vi "save_time_average.vi"(7 "stimulation type enum":T1, 8 "error in (no error)":errorcluster, 9 "base name":string, 10 "folder path":path, 11 "DataCollectionMG091001IntrinsicImaging in":refnum<class "DataCollectionMG091001IntrinsicImaging.lvclass">) -> (0 "error out":errorcluster, 3 "DataCollectionMG091001IntrinsicImaging out":refnum<class "DataCollectionMG091001IntrinsicImaging.lvclass">)   [LabVIEW 2010, in "DataCollectionMG091001IntrinsicImaging.lvclass"]
uses:
  DataCollectionMG091001IntrinsicImaging.lvclass
  sweep_part_enum.ctl
  common/classes/ImageCollection/ImageCollection/ImageCollection.lvclass
  DataCollectionMG091001IntrinsicImaging.lvclass/DataCollectionMG091001IntrinsicImaging.ctl
  common/classes/ImageCollection/ImageCollection/add_mode_enum.ctl
  common/classes/ErrorController/ErrorController/class_data.vi
  common/classes/ErrorController/ErrorController/ErrorController.lvclass
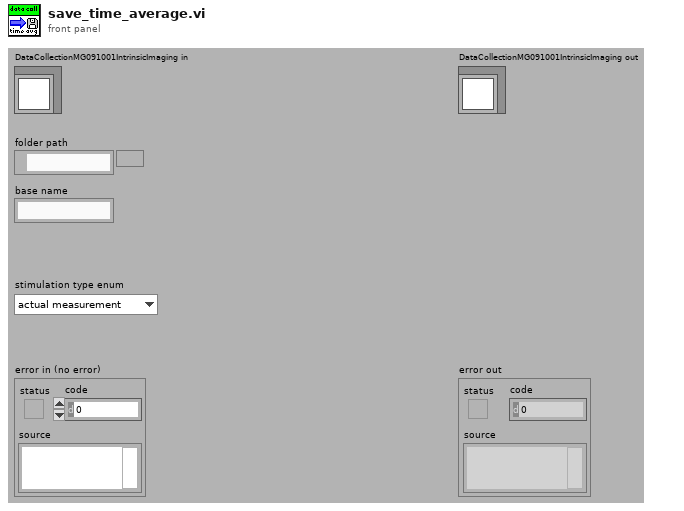
[diagram p1: front panel]
types:
  T1 = typedef "DataCollectionMG091001IntrinsicImaging.lvclass/sweep_part_enum.ctl" = enum16{"actual measurement", "control"}
  T2 = typedef "ImageCollection.lvclass/add_mode_enum.ctl" = enum16{"instance", "copy"}
  T3 = typedef "DataCollectionMG091001IntrinsicImaging.lvclass/individual_sweeps_saving_enum.ctl" = enum32{"autosave sweeps on the fly", "save individual sweeps", "don't save individual sweeps"}
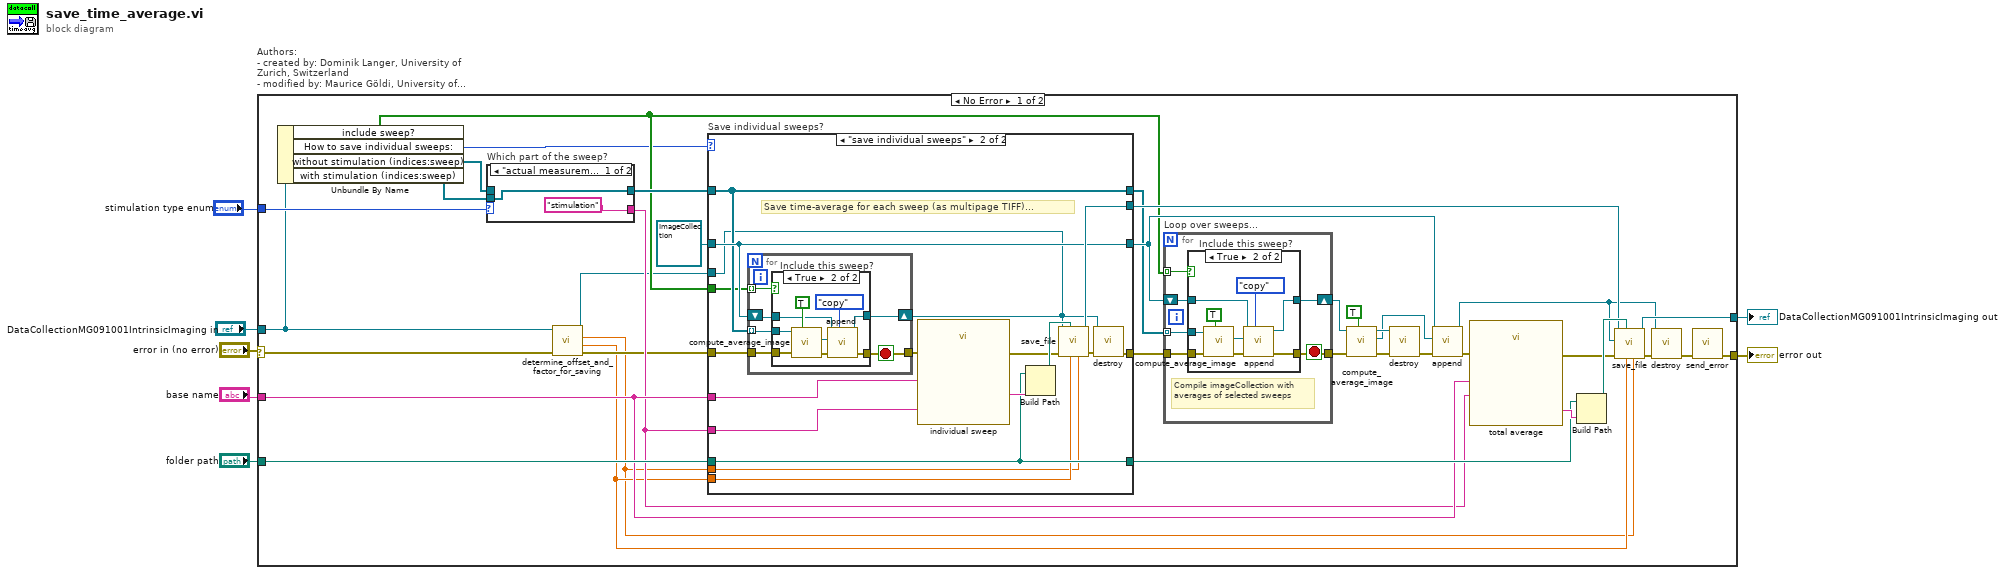
[diagram p0: block diagram]
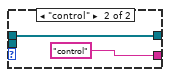
[diagram p2: hidden frame]
diagram:
  n1 = case "Authors: \n- created by: Dominik Langer, University of Zurich, Switzerland\n- modified by: Maurice Göldi, University of Zurich, Switzerland\n- modified by: Dominik Langer, University of Zurich, Switzerland" shown="No Error" "error in (no error)" {
    selector: "error in (no error)" -> [w15 w107]
    tunnel: [w16 w107] -> w6
    tunnel: [w44 w106] -> w4
    tunnel: "DataCollectionMG091001IntrinsicImaging in" -> [w13 w106]
    tunnel: "base name" -> [w26 _]
    tunnel: "folder path" -> [w43 _]
    tunnel: "stimulation type enum" -> [w22 _]
    frame No Error {
      n2 = Unbundle By Name(w13) -> ("include sweep?"=w19:bool[], "How to save individual sweeps:"=w18:T3, "without stimulation (indices:sweep)"=w23:refnum<class "ImageCollection.lvclass">[], "with stimulation (indices:sweep)"=w24:refnum<class "ImageCollection.lvclass">[])
      n3 = case "Which part of the sweep?" shown="\"actual measurement\", Default" w22 {
        tunnel: w23 -> [_ w48]
        tunnel: w24 -> [w46 _]
        tunnel: [w46 w48] -> w21
        tunnel: ["stimulation" "control"] -> w20
        frame "actual measurement", Default {
        }
        frame "control" {
        }
      }
      n4 = call-dynamic "determine_offset_and_factor_for_saving.vi"("error in (no error)"=w15, "DataCollectionMG091001IntrinsicImaging in"=w13) -> ("error out"=w14:errorcluster, "factor"=w9:dbl, "offset"=w8:dbl, "DataCollectionMG091001IntrinsicImaging out"=w12:refnum<class "DataCollectionMG091001IntrinsicImaging.lvclass">)  [unwired: 6 in]
      n5 = case "Save individual sweeps?" shown="\"save individual sweeps\"" w18 {
        tunnel: w14 -> [w70 w88]
        tunnel: w12 -> [w69 w75]
        tunnel: w21 -> [w66 w77]
        tunnel: [w69 w85] -> w29
        tunnel: w26 -> [_ w82]
        tunnel: w20 -> [_ w81]
        tunnel: w43 -> [w68 w79]
        tunnel: [w70 w80] -> w31
        tunnel: [w68 w79] -> w30
        tunnel: refnum<class "ImageCollection.lvclass"> refnum ("ImageCollection.lvclass") -> [w67 w78]
        tunnel: [w67 w78] -> w28
        tunnel: [w66 w77] -> w27
        tunnel: w19 -> [_ w76]
        tunnel: w9 -> [_ w72]
        tunnel: w8 -> [_ w71]
        frame Default {
        }
        frame "save individual sweeps" {
          # "Save time-average for each sweep (as multipage TIFF)..."
          n6 = for {
            tunnel: w77 -> [w94] mode=indexing
            shift-right: [w91] -> w73
            shift-left: w78 -> [w92]
            tunnel: w76 -> [w90] mode=indexing
            tunnel: w88 -> [w93]
            tunnel: [w89] -> w87
            stop <- w89 stop-if-true
            n7 = case "Include this sweep?" shown="True" w90 {
              tunnel: w94 -> [_ w105]
              tunnel: w93 -> [w96 w103]
              tunnel: w92 -> [w95 w101]
              tunnel: [w95 w99] -> w91
              tunnel: [w96 w97] -> w89
              frame False {
              }
              frame True {
                n8 = call-dynamic "compute_average_image.vi"("all?"=TRUE, "error in (no error)"=w103, "ImageCollection in"=w105) -> ("error out"=w102:errorcluster, "averaged image"=w100:refnum<class "Image.lvclass">)  [unwired: 6 in, 1 out]
                n9 = call-dynamic "append.vi"("add mode"=add_mode_enum."copy", "error in (no error)"=w102, "Image.lvclass"=w100, "ImageCollection in"=w101) -> ("error out"=w97:errorcluster, "ImageCollection out"=w99:refnum<class "ImageCollection.lvclass">)  [unwired: 5 in, 1 out]
              }
            }
          }
          n10 = call "individual sweep"("base"=w82, "type"=w81, "error in (no error)"=w87) -> ("Result"=w86:string, "error out"=w74:errorcluster)  [unwired: 11 in]
          n11 = Build Path(base path=w79, name or relative path=w86) -> (appended path=w84:path)
          n12 = call-dynamic "save_file.vi"("offset"=w71, "multiplication factor"=w72, "path"=w84, "error in (no error)"=w74, "ImageCollection in"=w73, "DataCollectionDL090215 in"=w75) -> ("error out"=w83:errorcluster, "DataCollectionDL090215 out"=w85:refnum<class "DataCollectionMG091001IntrinsicImaging.lvclass">)  [unwired: 4 in]
          n13 = call-dynamic "destroy.vi"("error in (no error)"=w83, "ImageCollection in"=w73) -> ("error out"=w80:errorcluster)  [unwired: 8 in, 1 out]
        }
      }
      n14 = for "Loop over sweeps..." {
        shift-right: [w52] -> w38
        shift-left: w28 -> [w53]
        tunnel: w19 -> [w50] mode=indexing
        tunnel: w27 -> [w51] mode=indexing
        tunnel: w31 -> [w54]
        tunnel: [w49] -> w42
        stop <- w49 stop-if-true
        # "Compile imageCollection with averages of selected sweeps"
        n15 = case "Include this sweep?" shown="True" w50 {
          tunnel: w54 -> [w56 w63]
          tunnel: [w56 w62] -> w49
          tunnel: w53 -> [w55 w59]
          tunnel: [w55 w58] -> w52
          tunnel: w51 -> [_ w57]
          frame False {
          }
          frame True {
            n16 = call-dynamic "compute_average_image.vi"("all?"=TRUE, "error in (no error)"=w63, "ImageCollection in"=w57) -> ("error out"=w65:errorcluster, "averaged image"=w60:refnum<class "Image.lvclass">)  [unwired: 6 in, 1 out]
            n17 = call-dynamic "append.vi"("add mode"=add_mode_enum."copy", "error in (no error)"=w65, "Image.lvclass"=w60, "ImageCollection in"=w59) -> ("error out"=w62:errorcluster, "ImageCollection out"=w58:refnum<class "ImageCollection.lvclass">)  [unwired: 5 in, 1 out]
          }
        }
      }
      n18 = call-dynamic "compute_average_image.vi"("all?"=TRUE, "error in (no error)"=w42, "ImageCollection in"=w38) -> ("error out"=w41:errorcluster, "averaged image"=w32:refnum<class "Image.lvclass">, "ImageCollection out"=w40:refnum<class "ImageCollection.lvclass">)  [unwired: 6 in]
      n19 = call-dynamic "destroy.vi"("error in (no error)"=w41, "ImageCollection in"=w40) -> ("error out"=w34:errorcluster)  [unwired: 8 in, 1 out]
      n20 = call-dynamic "append.vi"("error in (no error)"=w34, "Image.lvclass"=w32, "ImageCollection in"=w28) -> ("error out"=w33:errorcluster, "ImageCollection out"=w11:refnum<class "ImageCollection.lvclass">)  [unwired: 6 in, 1 out]
      n21 = call "total average"("base"=w26, "type"=w20, "error in (no error)"=w33) -> ("Result"=w37:string, "error out"=w10:errorcluster)  [unwired: 11 in]
      n22 = Build Path(base path=w30, name or relative path=w37) -> (appended path=w36:path)
      n23 = call-dynamic "save_file.vi"("offset"=w8, "multiplication factor"=w9, "path"=w36, "error in (no error)"=w10, "ImageCollection in"=w11, "DataCollectionDL090215 in"=w29) -> ("error out"=w35:errorcluster, "DataCollectionDL090215 out"=w44:refnum<class "DataCollectionMG091001IntrinsicImaging.lvclass">)  [unwired: 4 in]
      n24 = call-dynamic "destroy.vi"("error in (no error)"=w35, "ImageCollection in"=w11) -> ("error out"=w17:errorcluster)  [unwired: 8 in, 1 out]
      n25 = call "send_error.vi"("error in (no error)"=w17) -> ("error out"=w16:errorcluster)  [unwired: 10 in]
    }
    frame Error {
    }
  }
  "error out" <- w6
  "DataCollectionMG091001IntrinsicImaging out" <- w4
